vi "dui.vi"() -> ()   [LabVIEW 2018]
uses:
  <vilib>/Instr/_visa.llb/VISA Configure Serial Port (Instr).vi
panel:
  out "true 4":bool
  out "true 3":bool
  out "true 2":bool
  in  "OK Button 3":bool
  in  "OK Button 2":bool
  in  "OK Button":bool
  out "OK 2":bool caption="OK"
  out "OK":bool
  out "error out 2":errorcluster
  out "error out":errorcluster
  out "code out":i32 format="%0.0f"
  out "source out":string
  out "Which Button?":T1(ring)=enum."Center Button"
  out "T button?":bool
  out "true":bool
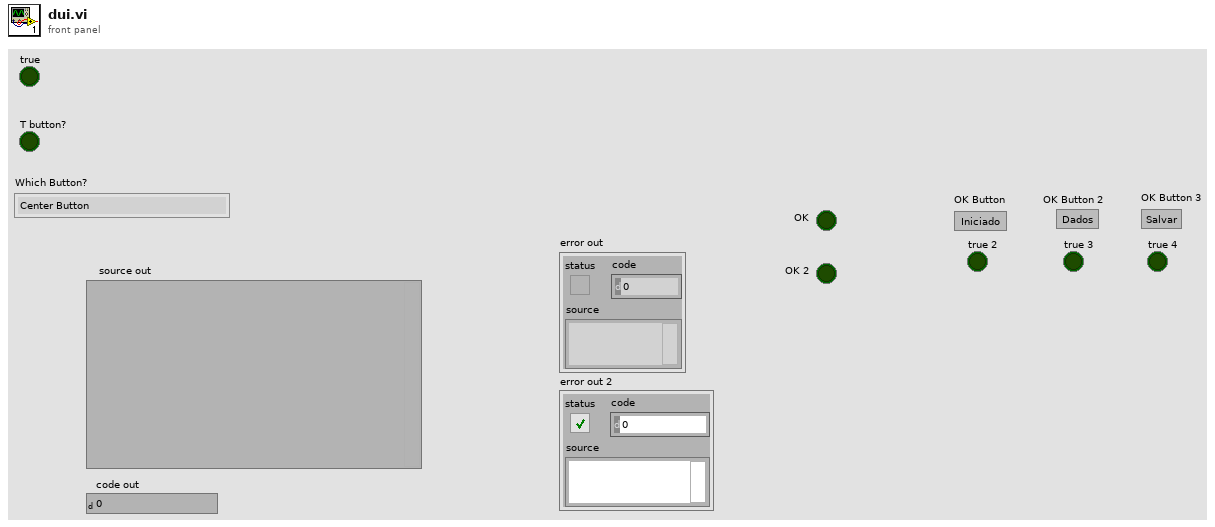
[diagram p1: front panel]
types:
  T1 = enum16{"Left Button", "Center Button", "Right Button", "Window Close"}
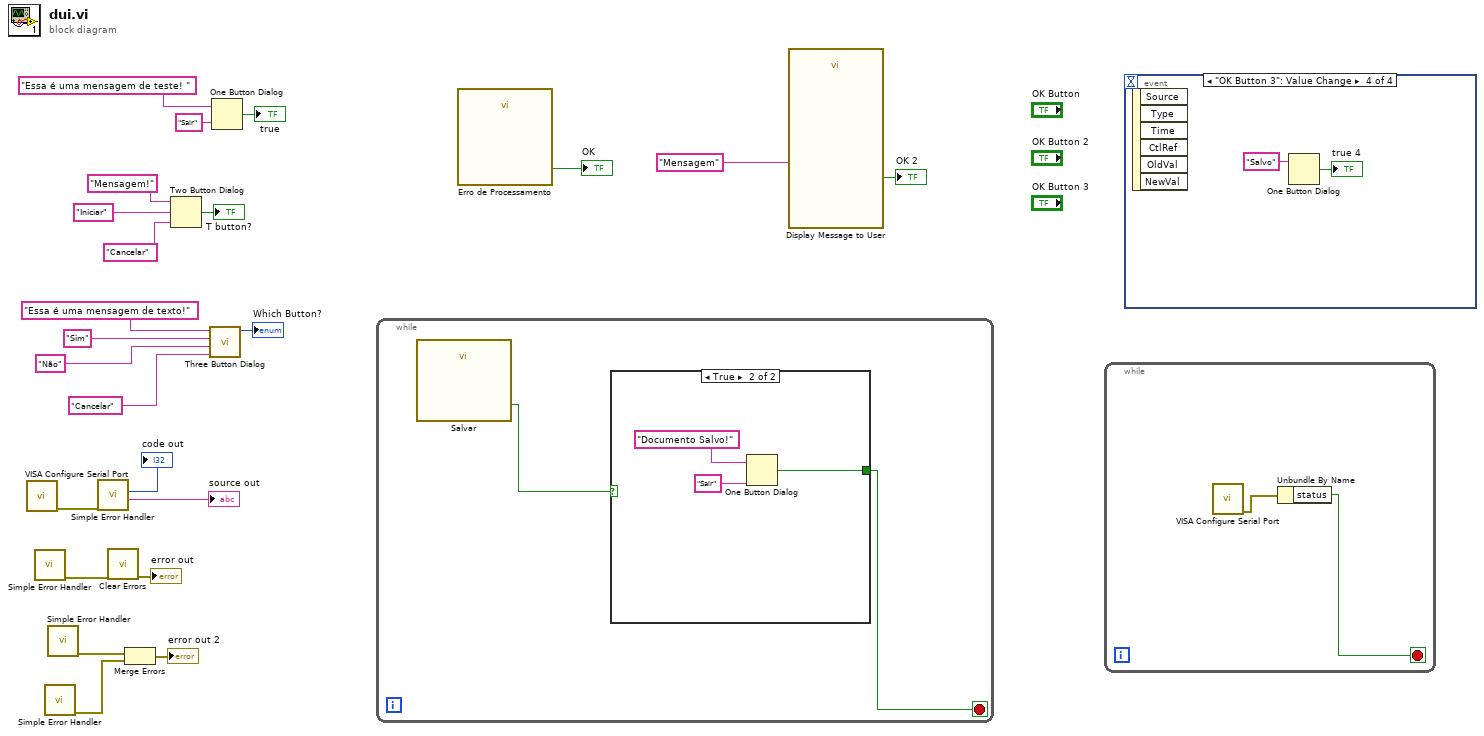
[diagram p0: block diagram]
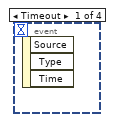
[diagram p2: hidden frame]
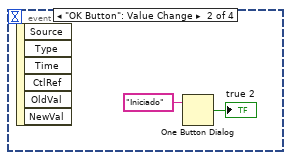
[diagram p3: hidden frame]
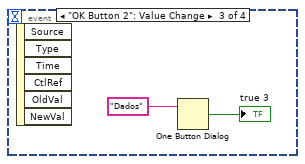
[diagram p4: hidden frame]
diagram:
  n1 = call-poly "VISA Configure Serial Port"() -> ("error out"=w11:errorcluster)  [unwired: 14 in, 1 out]
  n2 = call <vilib>:"Simple Error Handler.vi"() -> ("error out"=w8:errorcluster)  [unwired: 5 in, 4 out]
  n3 = call <vilib>:"Simple Error Handler.vi"() -> ("error out"=w5:errorcluster)  [unwired: 5 in, 4 out]
  n4 = call <vilib>:"Simple Error Handler.vi"() -> ("error out"=w6:errorcluster)  [unwired: 5 in, 4 out]
  n5 = call <vilib>:"Simple Error Handler.vi"("error in (no error)"=w11) -> ("code out"=→"code out":i32, "source out"=→"source out":string)  [unwired: 4 in, 3 out]
  n6 = call <vilib>:"Clear Errors.vi"("error in (no error)"=w8) -> ("error out"=→"error out":errorcluster)  [unwired: 5 in, 1 out]
  n7 = Merge Errors(w6, w5) -> (→"error out 2":errorcluster)
  n8 = Two Button Dialog(message="Mensagem!", 1:"Cancelar" ("F button name (\"Cancel\")"), 2:"Iniciar" ("T button name (\"OK\")")) -> (T button?=→"T button?":bool)
  n9 = call <vilib>:"Three Button Dialog.vi"("Right Button Text (\"Cancel\")"="Cancelar" ("Right Button Text (\"Cancel\")"), "Center Button Text (\"No\")"="Não" ("Center Button Text (\"No\")"), "Left Button Text (\"Yes\")"="Sim" ("Left Button Text (\"Yes\")"), "message"="Essa é uma mensagem de texto!") -> ("Which Button?"=→"Which Button?":T1)  [unwired: 7 in]
  n10 = One Button Dialog(message="Essa é uma mensagem de teste! ", button name ("OK")="Sair") -> (true=→"true":bool)
  n11 = while {
    stop <- w24 stop-if-true
    n12 = call "Salvar"() -> ("Sim"=w25:bool)  [unwired: 18 in, 1 out]
    n13 = case shown="True" w25 {
      tunnel: [_ w26] -> w24
      frame False {
      }
      frame True {
        n14 = One Button Dialog(message="Documento Salvo!", button name ("OK")="Sair") -> (true=w26:bool)
      }
    }
  }
  n15 = call "Erro de Processamento"() -> ("OK"=→"OK":bool)  [unwired: 18 in, 1 out]
  n16 = call "Display Message to User"("Message"="Mensagem") -> ("OK"=→"OK 2":bool)  [unwired: 9 in, 1 out]
  n17 = while {
    stop <- w29 stop-if-true
    n18 = call-poly "VISA Configure Serial Port"() -> ("error out"=w30:errorcluster)  [unwired: 14 in, 1 out]
    n19 = Unbundle By Name(w30) -> ("status"=w29:bool)
  }
  n20 = event shown="[3] \"OK Button 3\": Value Change" {
    selector: _ -> [_ _ _ _]
    dyn-events: _ -> [_ _ _ _]
    timeout: _ -> [_ _ _ _]
    event Timeout {
      n21 = event-data() -> ()  [unwired: 1 in, 3 out]
    }
    event "OK Button": Value Change {
      n22 = event-data() -> ()  [unwired: 1 in, 6 out]
      n23 = One Button Dialog(message="Iniciado") -> (true=→"true 2":bool)  [unwired: 1 in]
    }
    event "OK Button 2": Value Change {
      n24 = event-data() -> ()  [unwired: 1 in, 6 out]
      n25 = One Button Dialog(message="Dados") -> (true=→"true 3":bool)  [unwired: 1 in]
    }
    event "OK Button 3": Value Change {
      n26 = event-data() -> ()  [unwired: 1 in, 6 out]
      n27 = One Button Dialog(message="Salvo") -> (true=→"true 4":bool)  [unwired: 1 in]
    }
  }
